vi "Init.vi"(4 "Data Queue Names":string[](array[string]), 6 "Data Notifier Names":string[](array[string]), 7 "Name":string, 8 "error in (no error)":errorcluster, 10 "MSS":refnum<class "Measure and Stimulus Subsystems.lvclass">, 11 "Sample PI Control in":refnum<class "Sample PI Control.lvclass">) -> (0 "error out":errorcluster, 3 "Sample PI Control out":refnum<class "Sample PI Control.lvclass">)   [LabVIEW 2023, in "Sample PI Control.lvclass"]
uses:
  Sample PI Control.lvclass
  Sample PI Control.lvclass/Sample PI Control.ctl
  Task/Task Base/Task Base.lvclass
  Measure and Stimulus Subsystems/Measure and Stimulus Subsystems.lvclass
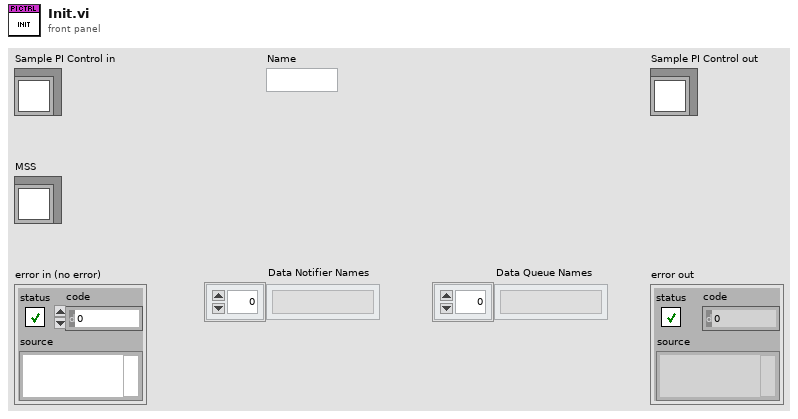
[diagram p1: front panel]
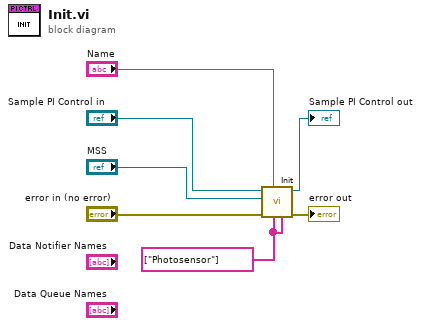
[diagram p0: block diagram]
diagram:
  w1 = string[] ["Photosensor"]
  n1 = call-parent "Init.vi"("Data Queue Names"=w1, "Data Notifier Names"=w1, "Name"="Name", "error in (no error)"="error in (no error)", "MSS"="MSS", "Task Base in"="Sample PI Control in") -> ("error out"=→"error out":errorcluster, "Task Base out"=→"Sample PI Control out":refnum<class "Sample PI Control.lvclass">)  [unwired: 4 in]
